vi "DMSV.get_CS_data.vi"(0 "csNotifiers":refnum<notifier>[][](array[refnum]), 5 "error in (no error)":errorcluster) -> (13 "lastUpdated":dbl[](array[numeric]), 14 "csNotifiers (out)":refnum<notifier>[][](array[refnum]), 15 "age":dbl[](array[numeric]), 16 "version":string[](array[string]), 18 "link?":bool[](array[boolean]), 19 "error out":errorcluster)   [LabVIEW 2014, in "DMSViewer.lvlib"]
doc: "Gets the DIM data of CS systems.\n\nauthor: Dietrich Beck, GSI\n\nLicense Agreement for this software:\n\nCopyright (C)\nGesellschaft für Schwerionenforschung, GSI\nPlanckstr. 1\n64291 Darmstadt\nGermany\n\nContact: D.Beck@gsi.de \n\nThis program is free software; you can redistribute it and/or modify it under the terms of the GNU General Public License as published by the Free Software Foundation; either version 2 of the license, or (at your option) any later version.\n\nThis program is distributed in the hope that it will be useful, but WITHOUT ANY WARRANTY; without even the implied warranty of MERCHANTABILITY or FITNESS FOR A PARTICULAR PURPOSE. See the GNU General License for more details (http://www.gnu.org).\n\nGesellschaft für Schwerionenforschung, GSI\nPlanckstr. 1, 64291 Darmstadt, Germany\nFor all questions and ideas contact: M.Richter@gsi.de, H.Brand@gsi.de or D.Beck@gsi.de.\nLast update: 10-OCT-2004"
uses:
  DMSViewer.lvlib
  CSlibraries-extern/DimLVEvent/LVDimInterface/LVDimInterface.lvlib
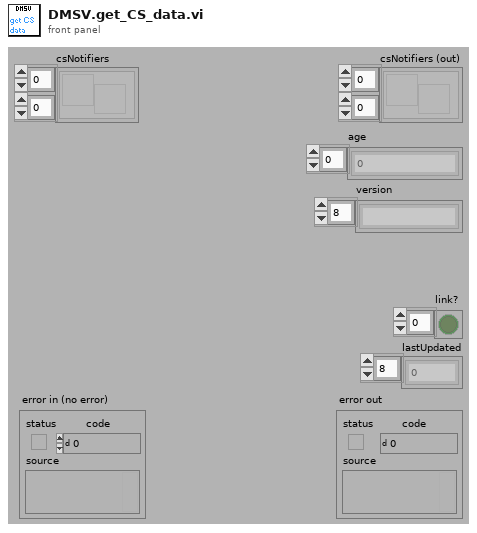
[diagram p1: front panel]
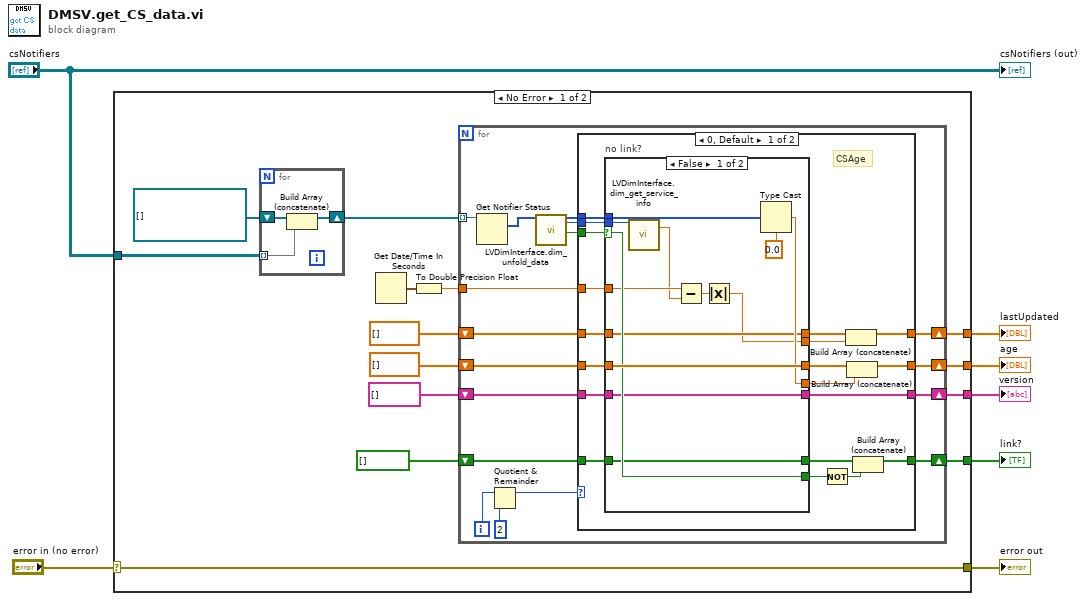
[diagram p0: block diagram]
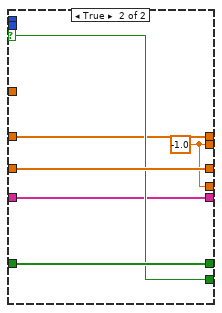
[diagram p2: hidden frame]
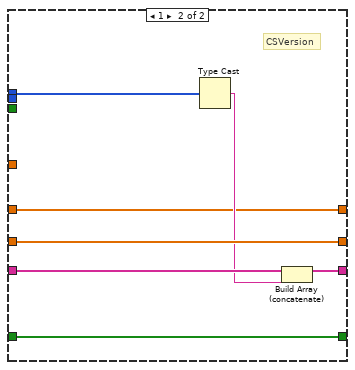
[diagram p3: hidden frame]
diagram:
  n1 = case shown="No Error" "error in (no error)" {
    selector: "error in (no error)" -> [w13 w87]
    tunnel: [w13 w87] -> w6
    tunnel: "csNotifiers" -> [w21 _]
    tunnel: [w14 _] -> w2
    tunnel: [w15 _] -> w3
    tunnel: [w16 _] -> w4
    tunnel: [w8 _] -> w1
    frame No Error {
      n2 = for {
        tunnel: w21 -> [w84] mode=indexing
        shift-right: [w86] -> w12
        shift-left: refnum<notifier>[] [] -> [w85]
        n3 = Build Array (concatenate)(w85, w84) -> (w86:refnum<notifier>[])
      }
      n4 = Get Date/Time In Seconds() -> (seconds since 1Jan1904=w11:timestamp)
      n5 = To Double Precision Float(number=w11) -> (double precision float=w9:dbl)
      n6 = for {
        shift-right: [w32] -> w14
        shift-left: dbl[] [] -> [w33]
        shift-right: [w30] -> w16
        shift-left: bool[] [] -> [w31]
        shift-right: [w28] -> w15
        shift-left: string[] [] -> [w29]
        tunnel: w12 -> [w27] mode=indexing
        shift-right: [w22] -> w8
        shift-left: dbl[] [] -> [w23]
        tunnel: w9 -> [w24]
        i -> [w38]
        n7 = Get Notifier Status(notifier=w27) -> (current notification=w26:i8[])  [unwired: 1 in, 4 out]
        n8 = Quotient & Remainder(x=w38, y=2) -> (x-y*floor(x/y)=w36:i32)  [unwired: 1 out]
        n9 = call "LVDimInterface.dim_unfold_data.vi"("rawData"=w26) -> ("data"=w35:i8[], "callBackID"=w25:i32, "no link"=w34:bool)  [unwired: 15 in, 1 out]
        n10 = case shown="0, Default" w36 {
          tunnel: w35 -> [w57 w83]
          tunnel: w34 -> [w46 _]
          tunnel: w33 -> [w56 w81]
          tunnel: [w53 w81] -> w32
          tunnel: w31 -> [w55 w78]
          tunnel: [w50 w78] -> w30
          tunnel: w29 -> [w48 w82]
          tunnel: [w47 w80] -> w28
          tunnel: w25 -> [w44 _]
          tunnel: w24 -> [w43 _]
          tunnel: w23 -> [w42 w77]
          tunnel: [w40 w77] -> w22
          frame 0, Default {
            # "CSAge"
            n11 = case "no link?" shown="False" w46 {
              selector: w46 -> [w66 w74]
              tunnel: w57 -> [w70 _]
              tunnel: w56 -> [w68 w76]
              tunnel: [w68 w76] -> w54
              tunnel: w55 -> [w65 w75]
              tunnel: [w67 w71] -> w52
              tunnel: [w66 w74] -> w49
              tunnel: [w65 w75] -> w51
              tunnel: [w64 w73] -> w47
              tunnel: w48 -> [w64 w73]
              tunnel: w44 -> [w63 _]
              tunnel: w43 -> [w62 _]
              tunnel: [w60 w72] -> w41
              tunnel: w42 -> [w60 w72]
              tunnel: [w58 w71] -> w39
              frame False {
                n12 = call "LVDimInterface.dim_get_service_info.vi"("callBackID"=w63) -> ("timeStamp"=w61:dbl)  [unwired: 9 in, 9 out]
                n13 = Subtract(x=w62, y=w61) -> (x-y=w59:dbl)
                n14 = Absolute Value(x=w59) -> (abs(x)=w58:dbl)
                n15 = Type Cast(type=0.0, x=w70) -> (*(type *) &x=w67:dbl)
              }
              frame True {
                w71 = -1.0
              }
            }
            n16 = Not(x=w49) -> (.not. x?=w45:bool)
            n17 = Build Array (concatenate)(w41, w39) -> (w40:dbl[])
            n18 = Build Array (concatenate)(w54, w52) -> (w53:dbl[])
            n19 = Build Array (concatenate)(w51, w45) -> (w50:bool[])
          }
          frame 1 {
            # "CSVersion"
            n20 = Type Cast(x=w83) -> (*(type *) &x=w79:string)  [unwired: 1 in]
            n21 = Build Array (concatenate)(w82, w79) -> (w80:string[])
          }
        }
      }
    }
    frame Error {
    }
  }
  "error out" <- w6
  "link?" <- w4
  "version" <- w3
  "age" <- w2
  "lastUpdated" <- w1
  "csNotifiers (out)" <- "csNotifiers"
